vi "Set Meta Data (TCP Ref).vi"(7 "meta data":T1[](array[typedef]), 8 "error in":errorcluster, 11 "connection ID":refnum<k5>) -> (0 "error out":errorcluster, 3 "connection info out":T2)   [LabVIEW 2013, in "NI STM.lvlib"]
doc: "Assigns the meta data cluster associated with this STM session."
uses:
  NI STM.lvlib
  TCP Connection Info.ctl
  SubVIs/MetaDataElement.ctl
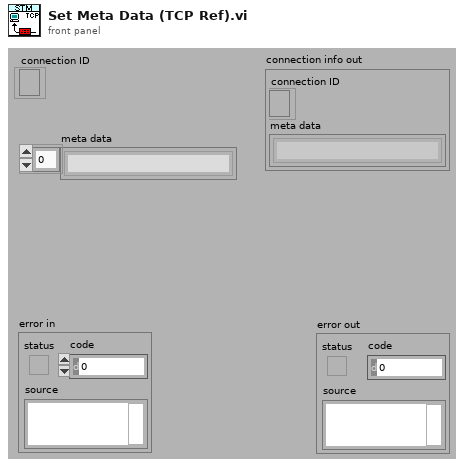
[diagram p1: front panel]
types:
  T1 = typedef "NI STM.lvlib/MetaDataElement.ctl" = string
  T2 = typedef "NI STM.lvlib/TCP Connection Info.ctl" = cluster{"connection ID":refnum<k5>, "meta data":T1[]}
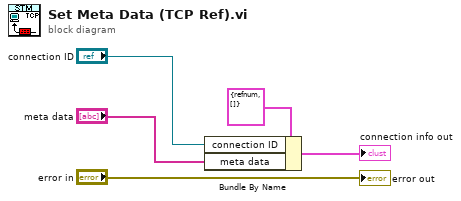
[diagram p0: block diagram]
diagram:
  n1 = Bundle By Name(cluster=T2 {"connection ID"=refnum, "meta data"=[]} ("Connection Info Out"), "connection ID"="connection ID", "meta data"="meta data") -> (→"connection info out":T2)
  "error out" <- "error in"
